vi "Update DUT Status.vi"(8 "error in (no error)":errorcluster, 11 "Module ID":i32=-1) -> (0 "error out":errorcluster)   [LabVIEW 2015, in "Device Under Test_Cloneable_DQMH.lvlib"]
doc: "Request Device Under Test to update the DUT status.\nBroadcast to any VI registered to listen to Device Under Test's broadcast events that the DUT Status was updated.\n_____\nCreated using Delacor QMH Event Scripter 1.0.0.50.\n____\nDelacor QMH Thermal Chamber Examples 4.0.0.21\nCopyright (c) 2018, Delacor"
uses:
  Device Under Test_Cloneable_DQMH.lvlib
  Update DUT Status Argument--cluster.ctl
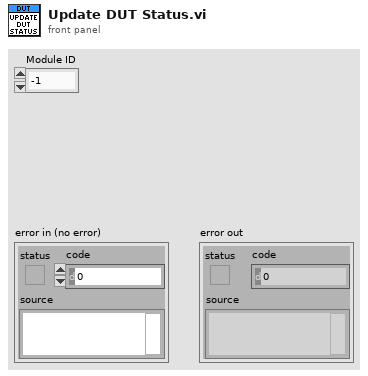
[diagram p1: front panel]
types:
  T1 = typedef "Device Under Test_Cloneable_DQMH.lvlib/Update DUT Status Argument--cluster.ctl" = cluster{"Module ID":i32, "Self Test Result":bool, "Power State":bool}
  T2 = typedef "Device Under Test_Cloneable_DQMH.lvlib/Request Events--cluster.ctl" = cluster{"Stop Module":refnum<user-event>, "Show Panel":refnum<user-event>, "Hide Panel":refnum<user-event>, "Show Diagram":refnum<user-event>, "Set Power State":refnum<user-event>, "Perform Self Test":refnum<user-event>, "Update DUT Status":refnum<user-event>, "Get Module Execution Status":refnum<user-event>}
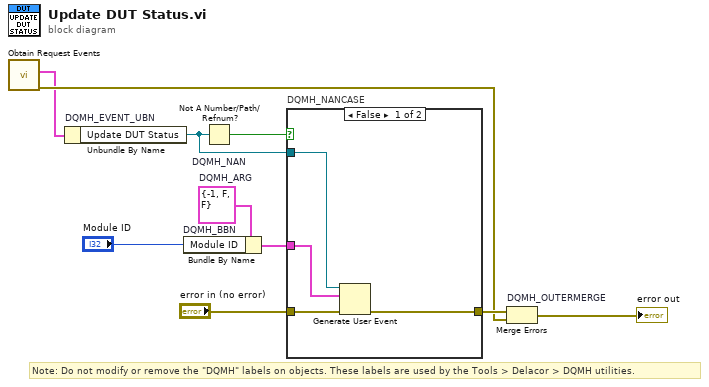
[diagram p0: block diagram]
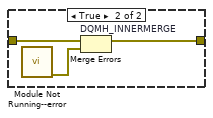
[diagram p2: hidden frame]
diagram:
  w4 = T1 {"Module ID"=-1, "Self Test Result"=FALSE, "Power State"=FALSE}  # DQMH_ARG
  # "Note: Do not modify or remove the \"DQMH\" labels on objects. These labels are used by the Tools > Delacor > DQMH utilities."
  n1 = call "Obtain Request Events.vi"() -> ("error out"=w2:errorcluster, "Device Under Test_Cloneable_DQMH Request Events"=w1:T2)  [unwired: 10 in]
  n2 = Unbundle By Name "DQMH_EVENT_UBN"(w1) -> ("Update DUT Status"=w5:refnum<user-event>)
  n3 = Bundle By Name "DQMH_BBN"(cluster=w4, "Module ID"="Module ID") -> (w7:T1)
  n4 = Not A Number/Path/Refnum? "DQMH_NAN"(number/path/refnum=w5) -> (NaN/Path/Refnum?=w6:bool)
  n5 = case "DQMH_NANCASE" shown="False" w6 {
    tunnel: "error in (no error)" -> [w14 w17]
    tunnel: [w13 w16] -> w8
    tunnel: w5 -> [w12 _]
    tunnel: w7 -> [w11 _]
    frame False {
      n6 = Generate User Event(user event=w12, event data cluster=w11, error in=w14) -> (error out=w13:errorcluster)  [unwired: 1 in, 1 out]
    }
    frame True {
      n7 = call "Module Not Running--error.vi"() -> ("error out"=w15:errorcluster)  [unwired: 11 in]
      n8 = Merge Errors "DQMH_INNERMERGE"(w17, w15) -> (w16:errorcluster)
    }
  }
  n9 = Merge Errors "DQMH_OUTERMERGE"(w8, w2) -> (→"error out":errorcluster)
